vi "Get Owning Project.vi"(7 "VI":refnum<vi>, 8 "error in":errorcluster) -> (0 "error out":errorcluster, 2 "Owning Project":refnum<vi>)   [LabVIEW 2024]
panel:
  out "Non-qualified Name":string
  out "VI Found":bool
  out "Project Name":string
  out "VI Name":string
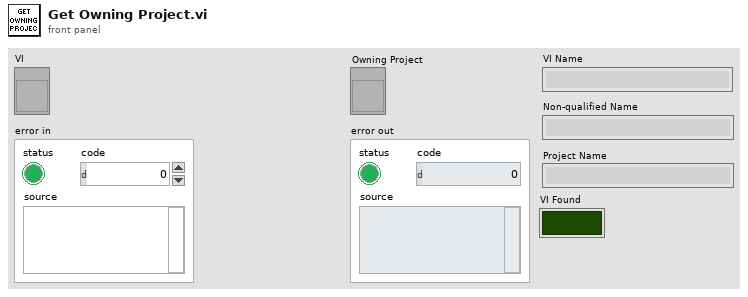
[diagram p1: front panel]
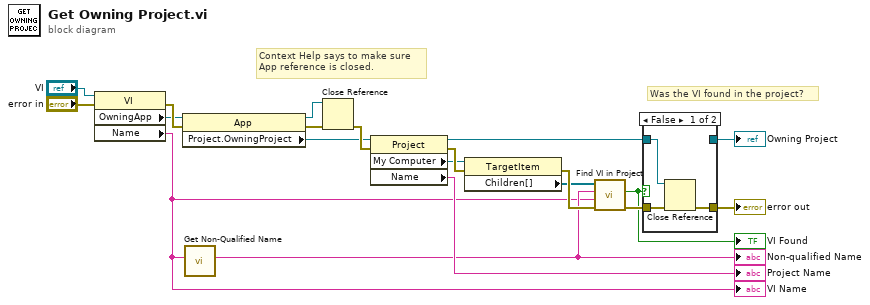
[diagram p0: block diagram]
diagram:
  # "Was the VI found in the project?"
  # "Context Help says to make sure App reference is closed."
  n1 = property class="VI"(reference="VI", error in="error in") -> (error out=w19:errorcluster, "OwningApp"=w10:refnum<vi>, "Name"=w1:string)  [unwired: 1 out]
  "VI Name" <- w1
  n2 = property class="App"(reference=w10, error in=w19) -> (reference out=w11:refnum<vi>, error out=w20:errorcluster, "Project.OwningProject"=w6:refnum<vi>)
  n3 = call "Get Non-Qualified Name.vi"("VI Name"=w1) -> ("Non-Qualified VI Name"=w2:string)  [unwired: 10 in]
  "Non-qualified Name" <- w2
  n4 = Close Reference(reference=w11, error in (no error)=w20) -> (error out=w15:errorcluster)
  n5 = property class="Project"(reference=w6, error in=w15) -> (reference out=w4:refnum<vi>, error out=w16:errorcluster, "My Computer"=w9:refnum<vi>, "Name"=→"Project Name":string)
  n6 = property class="TargetItem"(reference=w9, error in=w16) -> (error out=w17:errorcluster, "Children[]"=w7:refnum<vi>[])  [unwired: 1 out]
  n7 = call "Find VI in Project.vi"("error in"=w17, "VI Name"=w1, "Non-Qualified VI Name"=w2, "Project Items"=w7) -> ("error out"=w14:errorcluster, "VI Found"=w5:bool)  [unwired: 6 in]
  "VI Found" <- w5
  n8 = case shown="False" w5 {
    tunnel: w4 -> [w21 w24]
    tunnel: w14 -> [w23 w25]
    tunnel: [w22 w25] -> w13
    tunnel: [_ w24] -> w3
    frame False {
      n9 = Close Reference(reference=w21, error in (no error)=w23) -> (error out=w22:errorcluster)
    }
    frame True {
    }
  }
  "Owning Project" <- w3
  "error out" <- w13
